vi "Latch.vi"(10 "Input":bool) -> (3 "Boolean":bool)   [LabVIEW 2017]
panel:
  in  "Numeric":dbl
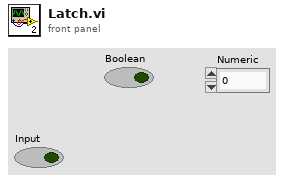
[diagram p1: front panel]
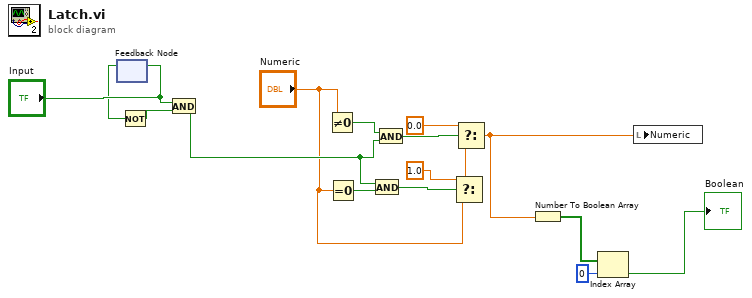
[diagram p0: block diagram]
diagram:
  n1 = feedback #1() -> (w4:bool)  [unwired: 1 in]
  n2 = feedback-in #1("Input") -> ()
  n3 = Not(x=w4) -> (.not. x?=w3:bool)
  n4 = And(x="Input", y=w3) -> (x .and. y?=w10:bool)
  n5 = Not Equal To 0?(x="Numeric") -> (x != 0?=w6:bool)
  n6 = Equal To 0?(x="Numeric") -> (x = 0?=w9:bool)
  n7 = And(x=w10, y=w9) -> (x .and. y?=w11:bool)
  n8 = And(x=w6, y=w10) -> (x .and. y?=w7:bool)
  n9 = Select(t=1.0, s=w11, f="Numeric") -> (s? t:f=w13:dbl)
  n10 = Select(t=0.0, s=w7, f=w13) -> (s? t:f=w2:dbl)
  n11 = Number To Boolean Array(number=w2) -> (Boolean array=w14:bool[])
  n12 = Index Array(array=w14, index=0) -> (element=→"Boolean":bool)
  n13 = local write "Numeric"(w2) -> ()
